vi "Filter Detected Signal.vi"(8 "error in (no error)":errorcluster, 11 "Software Lock-in in":refnum<class "Software Lock-in.lvclass">) -> (0 "error out":errorcluster, 3 "Software Lock-in out":refnum<class "Software Lock-in.lvclass">)   [LabVIEW 2020, in "Software Lock-in.lvclass"]
uses:
  Software Lock-in.lvclass
  Software Lock-in.lvclass/Software Lock-in.ctl
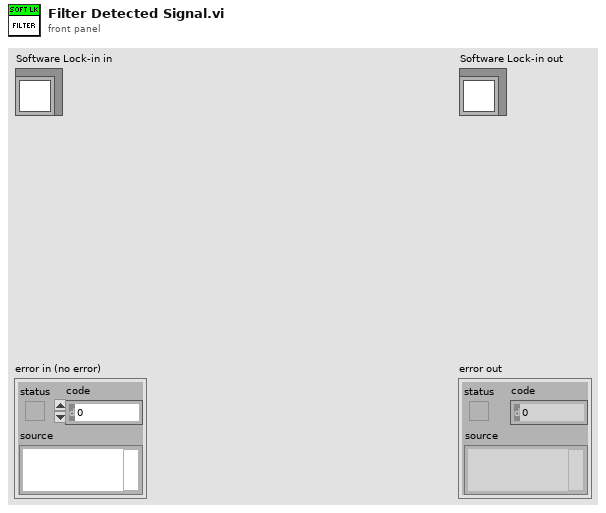
[diagram p1: front panel]
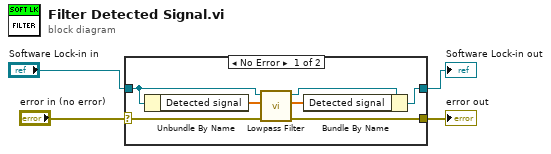
[diagram p0: block diagram]
diagram:
  n1 = case shown="No Error" "error in (no error)" {
    selector: "error in (no error)" -> [w9 w13]
    tunnel: [w10 w13] -> w3
    tunnel: [w11 w12] -> w1
    tunnel: "Software Lock-in in" -> [w8 w12]
    frame No Error {
      n2 = Unbundle By Name(w8) -> ("Detected signal"=w7:cdb[])
      n3 = call-dynamic "Lowpass Filter.vi"("error in (no error)"=w9, "Signal"=w7, "Lock-in Detector in"=w8) -> ("error out"=w10:errorcluster, "Signal out"=w6:cdb[], "Lock-in Detector out"=w5:refnum<class "Software Lock-in.lvclass">)  [unwired: 6 in]
      n4 = Bundle By Name(cluster=w5, "Detected signal"=w6) -> (w11:refnum<class "Software Lock-in.lvclass">)
    }
    frame Error {
    }
  }
  "error out" <- w3
  "Software Lock-in out" <- w1
